vi "Read Byte Stream.vi"(8 "error in (no error)":errorcluster, 11 "UTF8 in":refnum<class "UTF-8 String.lvclass">) -> (0 "error out":errorcluster, 2 "Byte Stream":T1, 3 "UTF8 out":refnum<class "UTF-8 String.lvclass">)   [LabVIEW 2019, in "JKI Unicode.lvlib" / "UTF-8 String.lvclass"]
doc: "JKI Unicode 1.0.0.7\nTomi Maila - JKI\nCopyright (c) 2016, JKI"
uses:
  UTF-8 String.lvclass
  Byte Stream.ctl
  UTF-8 String.lvclass/UTF-8 String.ctl
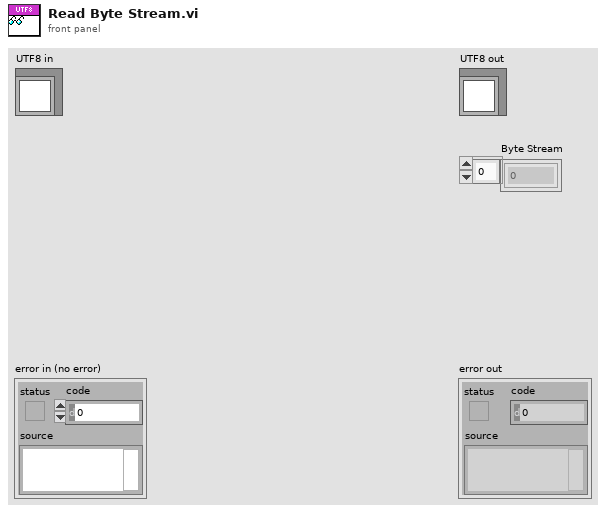
[diagram p1: front panel]
types:
  T1 = typedef "JKI Unicode.lvlib/UTF-8 String.lvclass/Byte Stream.ctl" = u8[]
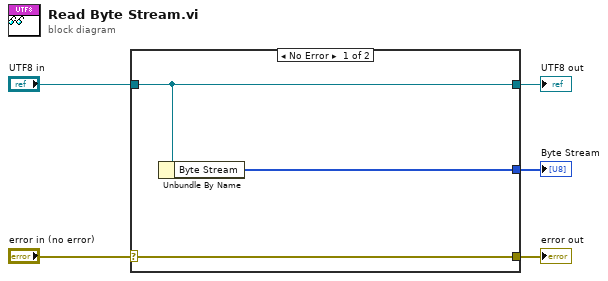
[diagram p0: block diagram]
diagram:
  n1 = case shown="No Error" "error in (no error)" {
    selector: "error in (no error)" -> [w8 w9]
    tunnel: [w8 w9] -> w4
    tunnel: [w7 w10] -> w2
    tunnel: "UTF8 in" -> [w7 w10]
    tunnel: [w6 _] -> w1
    frame No Error {
      n2 = Unbundle By Name(w7) -> ("Byte Stream"=w6:T1)
    }
    frame Error {
    }
  }
  "error out" <- w4
  "UTF8 out" <- w2
  "Byte Stream" <- w1
